vi "极化曲线.vi"(6 "Bool引用句柄":refnum<vi>, 8 "输出簇 3":T4, 9 "输出簇 2":T5, 10 "输出簇":T5, 11 "事件注册引用句柄 2":refnum<event-registration>) -> ()   [LabVIEW 2020]
uses:
  <vilib>/Utility/miscctls.llb/LVRectTypeDef.ctl
  Windows/System32/user32.dll
panel:
  in  "布尔 3":T1
  in  "布尔 2":T2
  in  "布尔":T3
  out "数值 2":dbl format="%#_2f V"
  out "数值":dbl format="%#_2f A"
  out "电流":dbl[](graph)
  out "电压":dbl[](graph)
  out "XY图":cluster{dbl[], dbl[]}(graph)
  # "极化曲线"
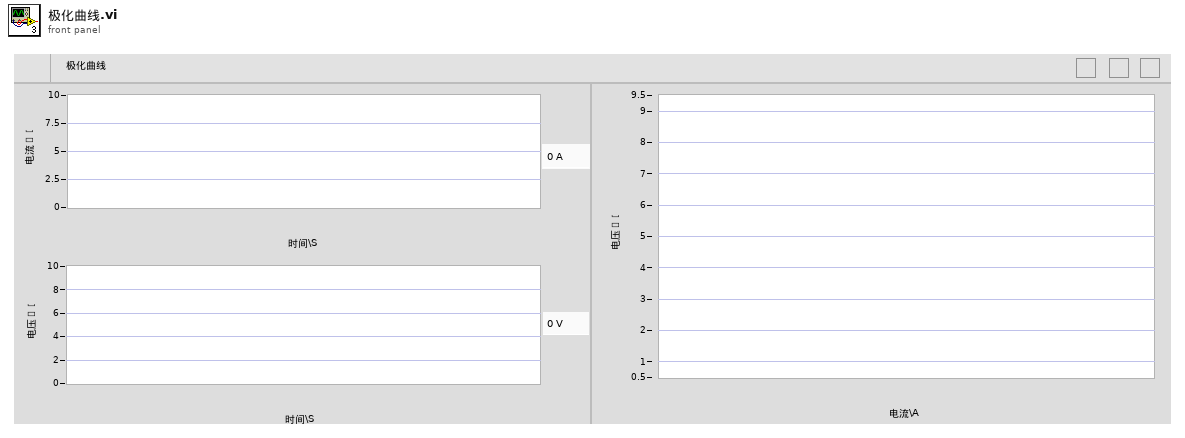
[diagram p1: front panel]
types:
  T1 = typedef "控件关闭.ctl" = bool
  T2 = typedef "控件最小化.ctl" = bool
  T3 = typedef "控件最大化.ctl" = bool
  T4 = cluster{"极化曲线1":refnum<vi>, "极化曲线2":refnum<vi>, "极化曲线3":refnum<vi>, "极化曲线4":refnum<vi>}
  T5 = cluster{"电流1":refnum<vi>, "电流2":refnum<vi>, "电流3":refnum<vi>, "电流4":refnum<vi>}
  T6 = typedef "LVRectTypeDef.ctl" = cluster{"Left":i16, "Top":i16, "Right":i16, "Bottom":i16}
  T7 = typedef "LVPoint32TypeDef.ctl" = cluster{"Horizontal":i32, "Vertical":i32}
  T8 = enum32{"Invalid", "Standard", "Closed", "Hidden", "Minimized", "Maximized"}
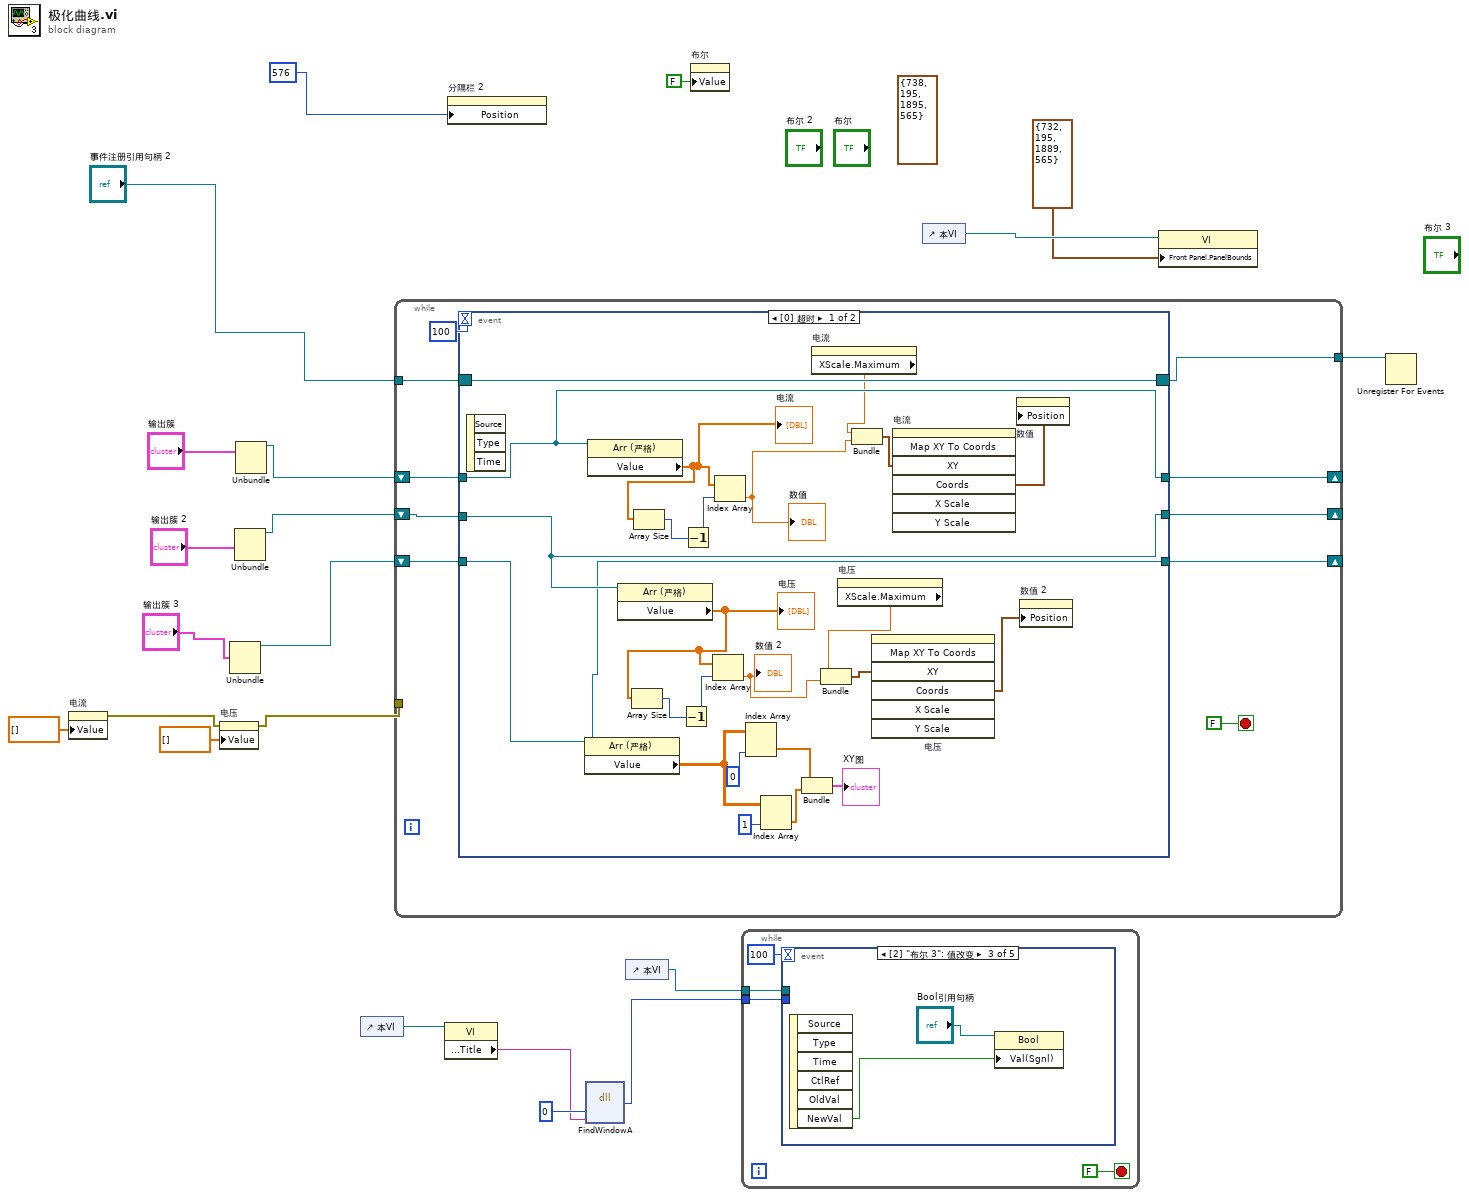
[diagram p0: block diagram]
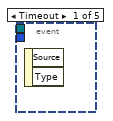
[diagram p2: hidden frame]
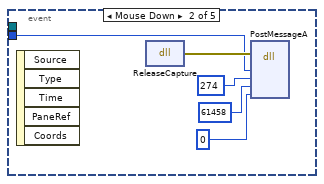
[diagram p3: hidden frame]
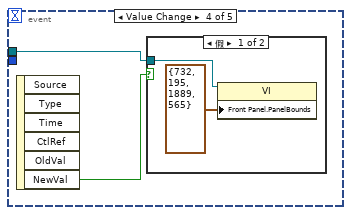
[diagram p4: hidden frame]
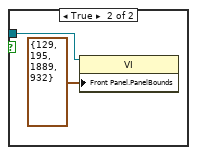
[diagram p5: hidden frame]
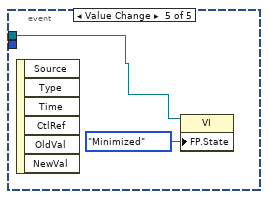
[diagram p6: hidden frame]
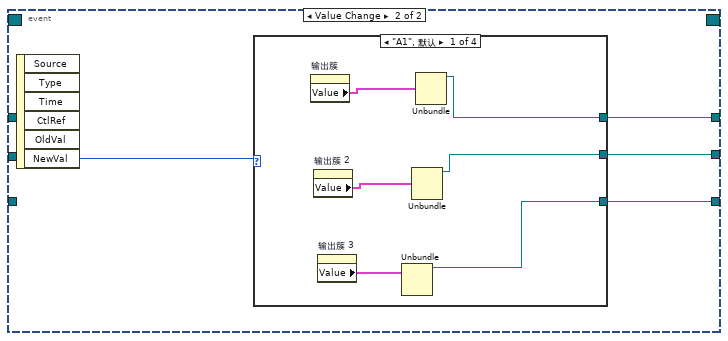
[diagram p7: hidden frame]
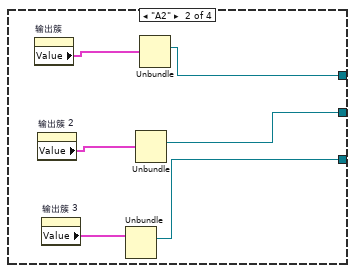
[diagram p8: hidden frame]
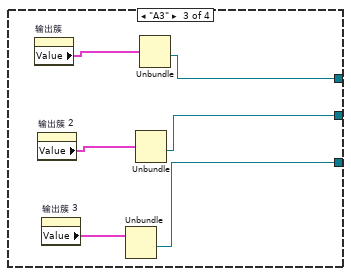
[diagram p9: hidden frame]
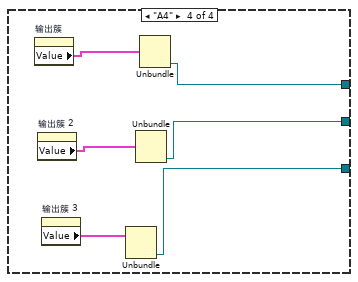
[diagram p10: hidden frame]
diagram:
  (unwired) T6 {"Left"=738, "Top"=195, "Right"=1895, "Bottom"=565} ("前面板窗口:前面板边界")
  n1 = property on="电流" class="WFGraph (严格)"("Value"=dbl[] [] ("电流")) -> (error out=w10:errorcluster)  [unwired: 2 in, 1 out]
  n2 = property on="电压" class="WFGraph (严格)"(error in=w10, "Value"=dbl[] [] ("电压")) -> (error out=w9:errorcluster)  [unwired: 1 in, 1 out]
  n3 = Unbundle("输出簇 3") -> ("极化曲线1"=w2:refnum<vi>)  [unwired: 3 out]
  n4 = Unbundle("输出簇 2") -> ("电流1"=w3:refnum<vi>)  [unwired: 3 out]
  n5 = Unbundle("输出簇") -> ("电流1"=w4:refnum<vi>)  [unwired: 3 out]
  n6 = control-ref of="本VI"() -> (w19:refnum<vi>)
  n7 = while {
    tunnel: w9 -> [_]
    tunnel: "事件注册引用句柄 2" -> [w30]
    tunnel: [w29] -> w8
    shift-right: [w28] -> _
    shift-left: w4 -> [w25]
    shift-right: [w27] -> _
    shift-left: w3 -> [w24]
    shift-right: [w26] -> _
    shift-left: w2 -> [w23]
    stop <- FALSE stop-if-true
    n8 = event shown="[0] 超时" {
      selector: w30 -> [w55 _]
      dyn-events: [w55 _] -> w29
      timeout: 100 -> [_ _]
      tunnel: [w52 w58] -> w28
      tunnel: [w51 w57] -> w27
      tunnel: [w50 w56] -> w26
      tunnel: w25 -> [w52 _]
      tunnel: w24 -> [w51 _]
      tunnel: w23 -> [w50 _]
      event Timeout {
        n9 = event-data() -> ()  [unwired: 1 in, 3 out]
        n10 = property class="Arr (严格)"(reference=w50) -> ("Value"=w49:dbl[][])  [unwired: 1 in, 2 out]
        n11 = property class="Arr (严格)"(reference=w52) -> ("Value"=w43:dbl[])  [unwired: 1 in, 2 out]
        "电流" <- w43
        n12 = property class="Arr (严格)"(reference=w51) -> ("Value"=w40:dbl[])  [unwired: 1 in, 2 out]
        "电压" <- w40
        n13 = Array Size(array=w40) -> (size(s)=w41:i32)
        n14 = Array Size(array=w43) -> (size(s)=w45:i32)
        n15 = Decrement(x=w41) -> (x-1=w42:i32)
        n16 = Decrement(x=w45) -> (x-1=w44:i32)
        n17 = Index Array(array=w40, index=w42) -> (element=w34:dbl)
        "数值 2" <- w34
        n18 = Index Array(array=w43, index=w44) -> (element=w38:dbl)
        "数值" <- w38
        n19 = Index Array(array=w49, index (col)=0 ("禁用的索引 (列)")) -> (element=w48:dbl[])  [unwired: 1 in]
        n20 = Index Array(array=w49, index (col)=1 ("禁用的索引 (列)")) -> (element=w47:dbl[])  [unwired: 1 in]
        n21 = Bundle("Value"=w48, "Value"=w47) -> (→"XY图":cluster{"Value":dbl[], "Value":dbl[]})  [unwired: 1 in]
        n22 = property on="电流" class="WFGraph (严格)"() -> ("XScale.Maximum"=w39:dbl)  [unwired: 2 in, 2 out]
        n23 = property on="电压" class="WFGraph (严格)"() -> ("XScale.Maximum"=w35:dbl)  [unwired: 2 in, 2 out]
        n24 = Bundle("XScale.Maximum"=w35, "数值"=w34) -> (w33:cluster{"XScale.Maximum":dbl, "数值":dbl})  [unwired: 1 in]
        n25 = Bundle("XScale.Maximum"=w39, "数值"=w38) -> (w37:cluster{"XScale.Maximum":dbl, "数值":dbl})  [unwired: 1 in]
        n26 = invoke on="电压" class="WFGraph (严格)" method="Map XY To Coords"("XY"=w33) -> ("Coords"=w32:T7)  [unwired: 6 in, 6 out]
        n27 = invoke on="电流" class="WFGraph (严格)" method="Map XY To Coords"("XY"=w37) -> ("Coords"=w36:T7)  [unwired: 6 in, 6 out]
        n28 = property on="数值" class="DigNum (严格)"("Position"=w36) -> ()  [unwired: 2 in, 2 out]
        n29 = property on="数值 2" class="DigNum (严格)"("Position"=w32) -> ()  [unwired: 2 in, 2 out]
      }
      event Value Change {
        n30 = event-data() -> ("NewVal"=w59:enum32{"未选择", "A1", "A2", "A3", "A4"})  [unwired: 1 in, 5 out]
        n31 = case shown="\"A1\", 默认" w59 {
          tunnel: [w62 w68 w74 w78] -> w58
          tunnel: [w61 w67 w73 w79] -> w57
          tunnel: [w60 w66 w72 w80] -> w56
          frame "A1", Default {
            n32 = property on="输出簇" class="Clust (严格)"() -> ("Value"=w65:T5)  [unwired: 2 in, 2 out]
            n33 = property on="输出簇 2" class="Clust (严格)"() -> ("Value"=w64:T5)  [unwired: 2 in, 2 out]
            n34 = property on="输出簇 3" class="Clust (严格)"() -> ("Value"=w63:T4)  [unwired: 2 in, 2 out]
            n35 = Unbundle(w63) -> ("极化曲线1"=w60:refnum<vi>)  [unwired: 3 out]
            n36 = Unbundle(w64) -> ("电流1"=w61:refnum<vi>)  [unwired: 3 out]
            n37 = Unbundle(w65) -> ("电流1"=w62:refnum<vi>)  [unwired: 3 out]
          }
          frame "A2" {
            n38 = property on="输出簇" class="Clust (严格)"() -> ("Value"=w71:T5)  [unwired: 2 in, 2 out]
            n39 = property on="输出簇 2" class="Clust (严格)"() -> ("Value"=w70:T5)  [unwired: 2 in, 2 out]
            n40 = property on="输出簇 3" class="Clust (严格)"() -> ("Value"=w69:T4)  [unwired: 2 in, 2 out]
            n41 = Unbundle(w69) -> ("极化曲线2"=w66:refnum<vi>)  [unwired: 3 out]
            n42 = Unbundle(w70) -> ("电流2"=w67:refnum<vi>)  [unwired: 3 out]
            n43 = Unbundle(w71) -> ("电流2"=w68:refnum<vi>)  [unwired: 3 out]
          }
          frame "A3" {
            n44 = property on="输出簇" class="Clust (严格)"() -> ("Value"=w77:T5)  [unwired: 2 in, 2 out]
            n45 = property on="输出簇 2" class="Clust (严格)"() -> ("Value"=w76:T5)  [unwired: 2 in, 2 out]
            n46 = property on="输出簇 3" class="Clust (严格)"() -> ("Value"=w75:T4)  [unwired: 2 in, 2 out]
            n47 = Unbundle(w75) -> ("极化曲线3"=w72:refnum<vi>)  [unwired: 3 out]
            n48 = Unbundle(w76) -> ("电流3"=w73:refnum<vi>)  [unwired: 3 out]
            n49 = Unbundle(w77) -> ("电流3"=w74:refnum<vi>)  [unwired: 3 out]
          }
          frame "A4" {
            n50 = property on="输出簇" class="Clust (严格)"() -> ("Value"=w83:T5)  [unwired: 2 in, 2 out]
            n51 = property on="输出簇 2" class="Clust (严格)"() -> ("Value"=w82:T5)  [unwired: 2 in, 2 out]
            n52 = property on="输出簇 3" class="Clust (严格)"() -> ("Value"=w81:T4)  [unwired: 2 in, 2 out]
            n53 = Unbundle(w81) -> ("极化曲线4"=w80:refnum<vi>)  [unwired: 3 out]
            n54 = Unbundle(w82) -> ("电流4"=w79:refnum<vi>)  [unwired: 3 out]
            n55 = Unbundle(w83) -> ("电流4"=w78:refnum<vi>)  [unwired: 3 out]
          }
        }
      }
    }
  }
  n56 = property class="VI"(reference=w19) -> ("Front Panel.Title"=w18:string)  [unwired: 1 in, 2 out]
  n57 = property on="分隔栏 2" class="Splitter"("Position"=576 ("分隔栏位置")) -> ()  [unwired: 2 in, 2 out]
  n58 = dll-call lib="/Windows/System32/user32.dll" fn="FindWindowA"("lp"=u32 0, "name"=w18) -> ("返回类型"=w16:u32)  [unwired: 5 in, 2 out]
  n59 = control-ref of="本VI"() -> (w13:refnum<vi>)
  n60 = property on="布尔" class="Bool (严格)"("Value"=T3 FALSE ("布尔")) -> ()  [unwired: 2 in, 2 out]
  n61 = while {
    tunnel: w16 -> [w87]
    tunnel: w13 -> [w86]
    stop <- FALSE stop-if-true
    n62 = event shown="[2] \"布尔 3\": 值改变" {
      selector: _ -> [_ _ _ _ _]
      dyn-events: _ -> [_ _ _ _ _]
      timeout: 100 -> [_ _ _ _ _]
      tunnel: w87 -> [_ w88 _ _ _]
      tunnel: w86 -> [_ _ _ w95 w102]
      event Timeout {
        n63 = event-data() -> ()  [unwired: 1 in, 2 out]
      }
      event Mouse Down {
        n64 = event-data() -> ()  [unwired: 1 in, 5 out]
        n65 = dll-call lib="/Windows/System32/user32.dll" fn="ReleaseCapture"() -> (error out=w92:errorcluster)  [unwired: 4 in, 1 out]
        n66 = dll-call lib="/Windows/System32/user32.dll" fn="PostMessageA"(error in=w92, "lp"=w88, "name"=274, "vak"=61458, "val"=0) -> ()  [unwired: 7 in, 2 out]
      }
      event Value Change {
        n67 = event-data() -> ("NewVal"=w93:T1)  [unwired: 1 in, 5 out]
        n68 = property class="Bool"(reference="Bool引用句柄", "Val(Sgnl)"=w93) -> ()  [unwired: 1 in, 2 out]
      }
      event Value Change {
        n69 = event-data() -> ("NewVal"=w96:T3)  [unwired: 1 in, 5 out]
        n70 = case shown="假" w96 {
          tunnel: w95 -> [w98 w100]
          frame False {
            n71 = property class="VI"(reference=w98, "Front Panel.PanelBounds"=T6 {"Left"=732, "Top"=195, "Right"=1889, "Bottom"=565} ("前面板窗口:前面板边界")) -> ()  [unwired: 1 in, 2 out]
          }
          frame True {
            n72 = property class="VI"(reference=w100, "Front Panel.PanelBounds"=T6 {"Left"=129, "Top"=195, "Right"=1889, "Bottom"=932} ("前面板窗口:前面板边界")) -> ()  [unwired: 1 in, 2 out]
          }
        }
      }
      event Value Change {
        n73 = event-data() -> ()  [unwired: 1 in, 6 out]
        n74 = property class="VI"(reference=w102, "FP.State"=T8."Minimized" ("前面板窗口:状态")) -> ()  [unwired: 1 in, 2 out]
      }
    }
  }
  n75 = control-ref of="本VI"() -> (w21:refnum<vi>)
  n76 = property class="VI"(reference=w21, "Front Panel.PanelBounds"=T6 {"Left"=732, "Top"=195, "Right"=1889, "Bottom"=565} ("前面板窗口:前面板边界")) -> ()  [unwired: 1 in, 2 out]
  n77 = Unregister For Events(event registration refnum=w8) -> ()  [unwired: 1 in, 1 out]
